vi "연속읽기응답(subVI).vi"(1 "응답프레임":string) -> (0 "Word 배열":u16[](array[numeric]))   [LabVIEW 2014]
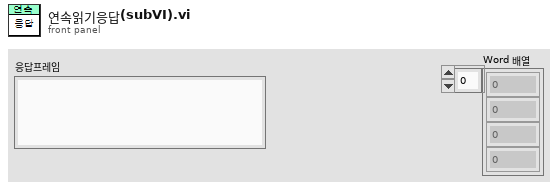
[diagram p1: front panel]
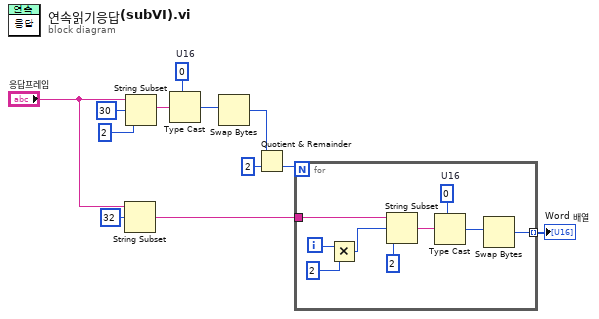
[diagram p0: block diagram]
diagram:
  w4 = u16 0  # U16
  n1 = String Subset(string="응답프레임", offset (0)=32 ("오프셋(0)")) -> (substring=w6:string)  [unwired: 1 in]
  n2 = String Subset(string="응답프레임", offset (0)=30 ("오프셋(0)"), length (rest)=2 ("길이(나머지)")) -> (substring=w5:string)
  n3 = Type Cast(type=w4, x=w5) -> (*(type *) &x=w3:u16)
  n4 = Swap Bytes(anything=w3) -> (byte swapped=w2:u16)
  n5 = Quotient & Remainder(x=w2, y=u16 2) -> (floor(x/y)=w7:u16)  [unwired: 1 out]
  n6 = for {
    N: w7 -> [_]
    tunnel: w6 -> [w21]
    tunnel: [w14] -> w1 mode=indexing
    i -> [w20]
    w16 = u16 0  # U16
    n7 = Multiply(x=w20, y=2) -> (x*y=w18:i32)
    n8 = String Subset(string=w21, offset (0)=w18, length (rest)=2 ("길이(나머지)")) -> (substring=w15:string)
    n9 = Type Cast(type=w16, x=w15) -> (*(type *) &x=w17:u16)
    n10 = Swap Bytes(anything=w17) -> (byte swapped=w14:u16)
  }
  "Word 배열" <- w1
